vi "clearpath_parse_firmware_info.vi"(0 "ClearpathComm":T1) -> (1 "Data Valid?":bool=TRUE, 2 "Write Time":u32 format="%x", 3 "Prot. Minor Ver.":u8, 4 "Prot. Major Ver.":u8, 5 "F/W Minor Ver.":u8, 6 "F/W Major Ver.":u8)   [LabVIEW 2012, in "clearpath_interface.lvlib"]
doc: "Parses firmware information as returned by platform. (Message type 0x8003)"
uses:
  clearpath_interface.lvlib
  cwrap_crio.dll
panel:
  # "Firmware Info"
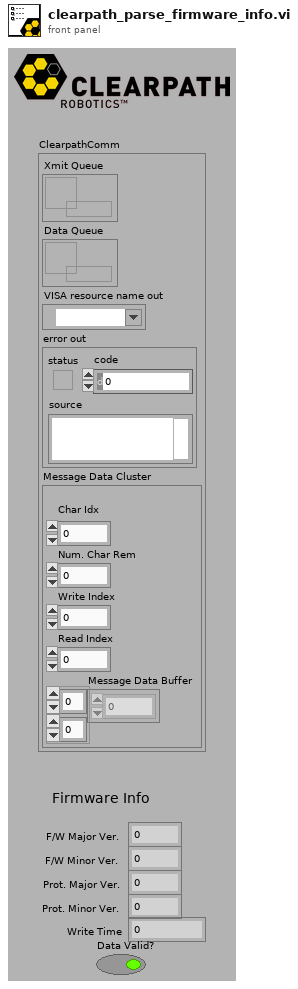
[diagram p1: front panel]
types:
  T1 = cluster{"Xmit Queue":refnum<queue>, "Data Queue":refnum<queue>, "VISA resource name out":refnum<visa-resource-name>, "error out":errorcluster, "Message Data Cluster":cluster{"\nChar Idx":u8, "Num. Char Rem":u8, "Write Index":u8, "Read Index":u8, "Message Data Buffer":u8[][]}}
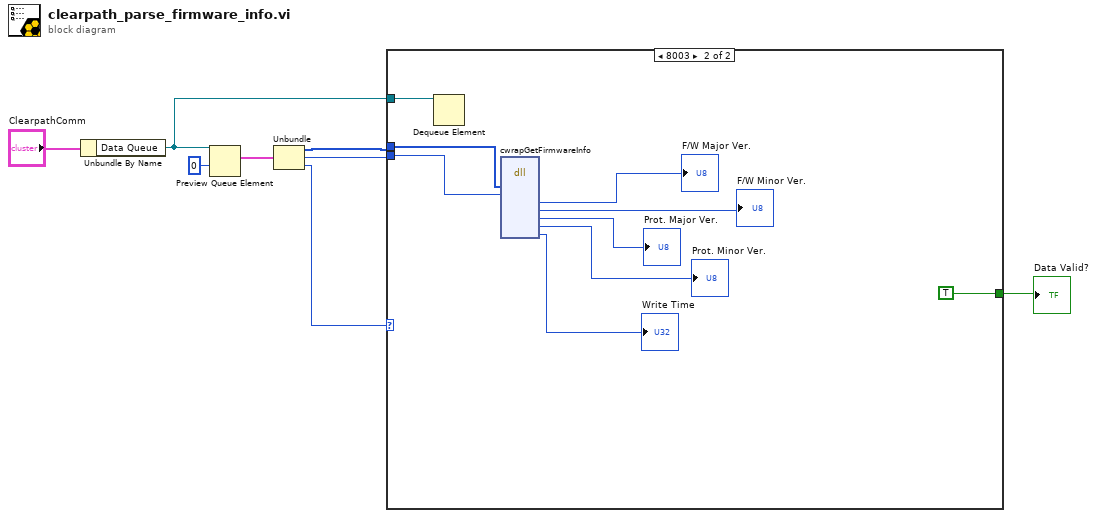
[diagram p0: block diagram]
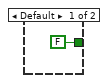
[diagram p2: hidden frame]
diagram:
  n1 = Unbundle By Name("ClearpathComm") -> ("Data Queue"=w1:refnum<queue>)
  n2 = Preview Queue Element(queue=w1, timeout in ms (-1)=0) -> (element=w6:cluster{u8[], "Length":i32, "Type":i32})  [unwired: 1 in, 3 out]
  n3 = Unbundle(w6) -> (w3:u8[], "Length"=w4:i32, "Type"=w5:i32)
  n4 = case shown="8003" w5 {
    tunnel: w4 -> [_ w12]
    tunnel: w3 -> [_ w13]
    tunnel: [FALSE TRUE] -> w2
    tunnel: w1 -> [_ w10]
    frame Default {
    }
    frame 32771 {
      n5 = Dequeue Element(queue=w10) -> ()  [unwired: 2 in, 4 out]
      n6 = dll-call lib="C:/Users/tebbeam/Documents/GitHub/IGVC-2013/Code/Project 1.0/Motors/Husky/cwrap_cRIO.*" fn="cwrapGetFirmwareInfo"("packet"=w13, "len"=w12) -> ("firm_maj"=→"F/W Major Ver.":u8, "firm_min"=→"F/W Minor Ver.":u8, "proto_maj"=→"Prot. Major Ver.":u8, "proto_min"=→"Prot. Minor Ver.":u8, "wr_time"=→"Write Time":u32)  [unwired: 11 in, 2 out]
    }
  }
  "Data Valid?" <- w2
